vi "Near Line.vi"(9 "Line":T1, 10 "How Near?":i32=3, 11 "Brick Wall in":refnum<class "Brick Wall.lvclass">) -> (3 "Near Line":bool)   [LabVIEW 2015, in "Brick Wall.lvclass"]
uses:
  Brick Wall.lvclass
  Type Defs/Direction Enum.ctl
  Brick Wall.lvclass/Brick Wall.ctl
  Square/Board Size.vi
  SubVIs/Read-Only Globals.vi
  Common/Common.lvlib
  Type Defs/SB Type Defs.lvlib
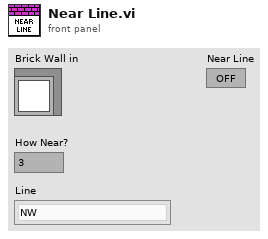
[diagram p1: front panel]
types:
  T1 = typedef "SB Type Defs.lvlib/Direction Enum.ctl" = enum16{"NW", "N", "NE", "E", "SE", "S", "SW", "W"}
  T2 = typedef "Common.lvlib/Position.ctl" = cluster{"Column":i32, "Row":i32}
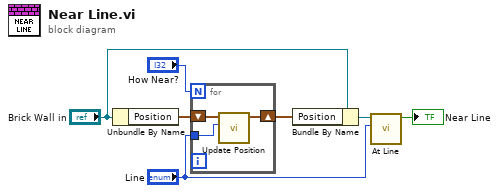
[diagram p0: block diagram]
diagram:
  n1 = Unbundle By Name("Brick Wall in") -> ("Position"=w2:T2)
  n2 = for {
    N: "How Near?" -> [_]
    tunnel: "Line" -> [w8]
    shift-right: [w9] -> w3
    shift-left: w2 -> [w10]
    n3 = call "Update Position.vi"("Direction"=w8, "Position in"=w10) -> ("Position out"=w9:T2)  [unwired: 9 in]
  }
  n4 = Bundle By Name(cluster="Brick Wall in", "Position"=w3) -> (w4:refnum<class "Brick Wall.lvclass">)
  n5 = call "At Line.vi"("Line"="Line", "Brick Wall in"=w4) -> ("At Line"=→"Near Line":bool)  [unwired: 9 in]
